vi "Clear Cache.vi"(8 "error in (no error)":errorcluster, 11 "Unit Of Work in":refnum<class "Unit Of Work Session.lvclass">) -> (0 "error out":errorcluster)   [LabVIEW 2020, in "Conditu2.lvlib" / "Unit Of Work Session.lvclass"]
uses:
  Unit Of Work Session.lvclass
  Entity Class Map.ctl
  Entity ID.ctl
  Entity/Entity.lvclass
  Unit Of Work Session.lvclass/Unit Of Work Session.ctl
  Conditu2.lvlib
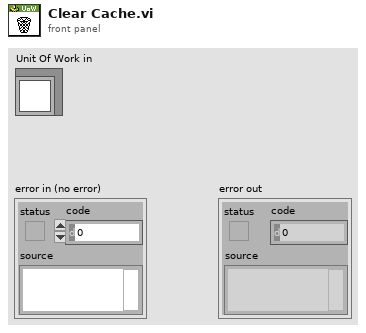
[diagram p1: front panel]
types:
  T1 = typedef "Conditu2.lvlib/Unit Of Work Session.lvclass/Entity Class Map.ctl" = map{string, map{T2, refnum<class "Entity.lvclass">}}
  T2 = typedef "Conditu2.lvlib/Entity ID.ctl" = i64
  T3 = typedef "Conditu2.lvlib/Unit Of Work Session.lvclass/Ref Data.ctl" = cluster{"Entity Class Map":T1}
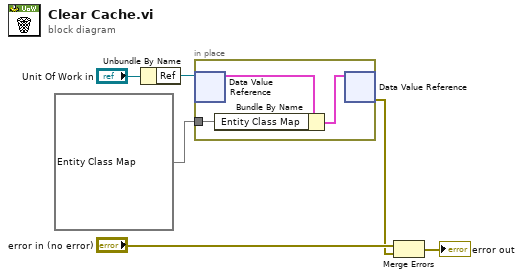
[diagram p0: block diagram]
diagram:
  n1 = Unbundle By Name("Unit Of Work in") -> ("Ref"=w5:refnum<data-value>)
  n2 = in-place {
    in-place-border: T1 {} ("Entity Class Map") -> [w7]
    n3 = in-place-dvr #1(w5) -> (w9:T3)  [unwired: 1 out]
    n4 = Bundle By Name(cluster=w9, "Entity Class Map"=w7) -> (w8:T3)
    n5 = in-place-dvr #1(w8) -> (w1:errorcluster)  [unwired: 1 out]
  }
  n6 = Merge Errors("error in (no error)", w1) -> (→"error out":errorcluster)
